vi "VI Tree.vi"   [LabVIEW 2012, in "Fluke 5080.lvlib"]
doc: "This is the instrument driver for the Fluke 5080A. The VI Tree displays all the user-callable VIs of the instrument driver in an organized table."
uses:
  <instrlib>/Fluke 5080/Fluke 5080.lvlib
panel:
  # "(c) 2010 National Instruments.  ALL RIGHTS RESERVED."
  # "SEE DIAGRAM\nFOR VI TREE."
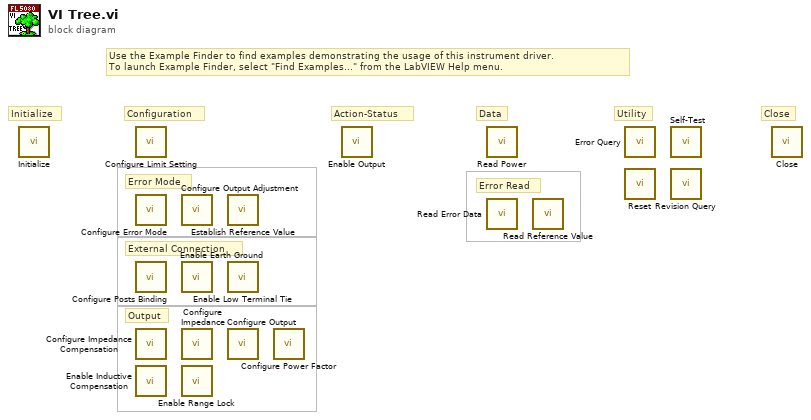
[diagram p0: block diagram]
diagram:
  # "Configuration"
  # "Close"
  # "Utility"
  # "Error Read"
  # "Data"
  # "Output"
  # "External Connection"
  # "Error Mode"
  # "Action-Status"
  # "Initialize"
  # "Use the Example Finder to find examples demonstrating the usage of this instrument driver.\nTo launch Example Finder, select \"Find Examples...\" from the LabVIEW Help menu."
  n1 = call <instrlib>:"Initialize.vi"() -> ()  [unwired: 10 in, 2 out]
  n2 = call <instrlib>:"Configure Limit Setting.vi"() -> ()  [unwired: 10 in, 2 out]
  n3 = call <instrlib>:"Configure Error Mode.vi"() -> ()  [unwired: 10 in, 2 out]
  n4 = call <instrlib>:"Configure Posts Binding.vi"() -> ()  [unwired: 10 in, 2 out]
  n5 = call <instrlib>:"Configure Impedance Compensation.vi"() -> ()  [unwired: 10 in, 2 out]
  n6 = call <instrlib>:"Enable Inductive Compensation.vi"() -> ()  [unwired: 10 in, 2 out]
  n7 = call <instrlib>:"Configure Output Adjustment.vi"() -> ()  [unwired: 10 in, 2 out]
  n8 = call <instrlib>:"Enable Earth Ground.vi"() -> ()  [unwired: 10 in, 2 out]
  n9 = call <instrlib>:"Configure Impedance.vi"() -> ()  [unwired: 10 in, 2 out]
  n10 = call <instrlib>:"Enable Range Lock.vi"() -> ()  [unwired: 10 in, 2 out]
  n11 = call <instrlib>:"Establish Reference Value.vi"() -> ()  [unwired: 10 in, 2 out]
  n12 = call <instrlib>:"Enable Low Terminal Tie.vi"() -> ()  [unwired: 10 in, 2 out]
  n13 = call <instrlib>:"Configure Output.vi"() -> ()  [unwired: 14 in, 2 out]
  n14 = call <instrlib>:"Configure Power Factor.vi"() -> ()  [unwired: 10 in, 2 out]
  n15 = call <instrlib>:"Enable Output.vi"() -> ()  [unwired: 10 in, 2 out]
  n16 = call <instrlib>:"Read Power.vi"() -> ()  [unwired: 9 in, 3 out]
  n17 = call <instrlib>:"Read Error Data.vi"() -> ()  [unwired: 8 in, 4 out]
  n18 = call <instrlib>:"Read Reference Value.vi"() -> ()  [unwired: 8 in, 4 out]
  n19 = call <instrlib>:"Error Query.vi"() -> ()  [unwired: 8 in, 4 out]
  n20 = call <instrlib>:"Reset.vi"() -> ()  [unwired: 10 in, 2 out]
  n21 = call <instrlib>:"Self-Test.vi"() -> ()  [unwired: 8 in, 4 out]
  n22 = call <instrlib>:"Revision Query.vi"() -> ()  [unwired: 8 in, 4 out]
  n23 = call <instrlib>:"Close.vi"() -> ()  [unwired: 11 in, 1 out]
